vi "initXY.vi"(0 "System no.":i32=1 min=1 step=1, 1 "xIdx":i32, 2 "yIdx":i32) -> (3 "xPos":dbl, 4 "yPos":dbl, 5 "xLim":dbl, 6 "yLim":dbl)   [LabVIEW 2015]
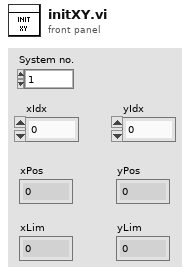
[diagram p1: front panel]
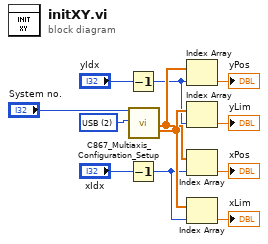
[diagram p0: block diagram]
diagram:
  w12 = u16 2 items=["RS232", "RS232 DaisyChain", "USB", "USB DaisyChain"] ("Interface")
  n1 = Decrement(x="yIdx") -> (x-1=w1:i32)
  n2 = Decrement(x="xIdx") -> (x-1=w4:i32)
  n3 = call "C867_Multiaxis_Configuration_Setup.vi"("System no."="System no.", "Interface"=w12) -> ("Position"=w9:dbl[], "+/- movement\nrange"=w10:dbl[])  [unwired: 11 in, 5 out]
  n4 = Index Array(array=w9, index=w1) -> (element=→"yPos":dbl)
  n5 = Index Array(array=w10, index=w1) -> (element=→"yLim":dbl)
  n6 = Index Array(array=w9, index=w4) -> (element=→"xPos":dbl)
  n7 = Index Array(array=w10, index=w4) -> (element=→"xLim":dbl)
